vi "Limits 2 Slider Values.vi"(9 "Actual":dbl[](array[numeric]), 10 "Offsets":dbl[](array[numeric]), 11 "Limits":T2) -> (2 "Values":T1(array[cluster]))   [LabVIEW 2009]
uses:
  Control Loop/Limit Matrix.ctl
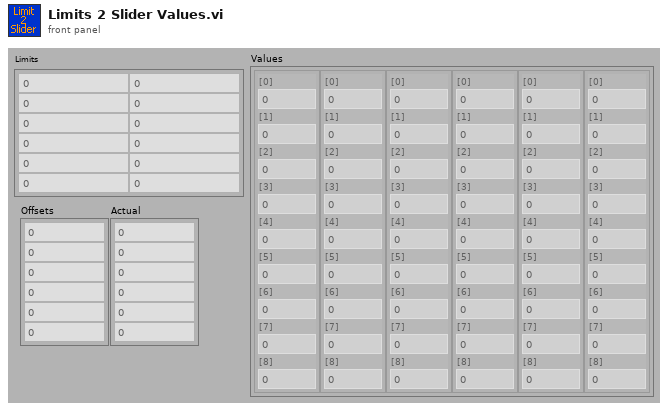
[diagram p1: front panel]
types:
  T1 = cluster{"[0]":dbl, "[1]":dbl, "[2]":dbl, "[3]":dbl, "[4]":dbl, "[5]":dbl, "[6]":dbl, "[7]":dbl, "[8]":dbl}[]
  T2 = typedef "Limit Matrix.ctl" = dbl[][]
  T3 = cluster{"[0]":dbl, "[1]":dbl, "[2]":dbl, "[3]":dbl, "[4]":dbl, "[5]":dbl, "[6]":dbl, "[7]":dbl, "[8]":dbl}
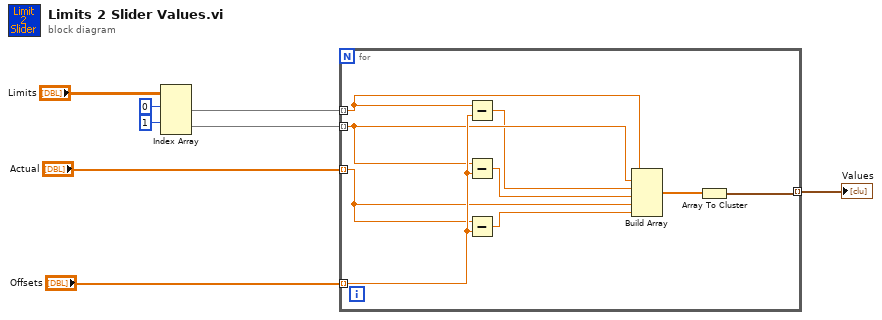
[diagram p0: block diagram]
diagram:
  n1 = Index Array(array="Limits", index (row) #1=0 ("index (row)"), index (row) #2=1 ("index (row)")) -> (element #1=w5:dbl[], element #2=w4:dbl[])  [unwired: 2 in]
  n2 = for {
    tunnel: w5 -> [w16] mode=indexing
    tunnel: w4 -> [w15] mode=indexing
    tunnel: "Actual" -> [w12] mode=indexing
    tunnel: "Offsets" -> [w17] mode=indexing
    tunnel: [w9] -> w1 mode=indexing
    n3 = Subtract(x=w16, y=w17) -> (x-y=w14:dbl)
    n4 = Subtract(x=w15, y=w17) -> (x-y=w13:dbl)
    n5 = Subtract(x=w12, y=w17) -> (x-y=w11:dbl)
    n6 = Build Array(w16, w15, w14, w13, w12, w11) -> (w10:dbl[])
    n7 = Array To Cluster(array=w10) -> (cluster=w9:T3)
  }
  "Values" <- w1
